vi "Read firmware file.vi"(2 "error in":errorcluster, 3 "RBF file path in":path) -> (0 "error out":errorcluster, 1 "firmware data":u8[](array[numeric]))   [LabVIEW 2013]
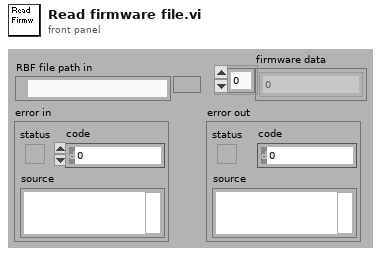
[diagram p1: front panel]
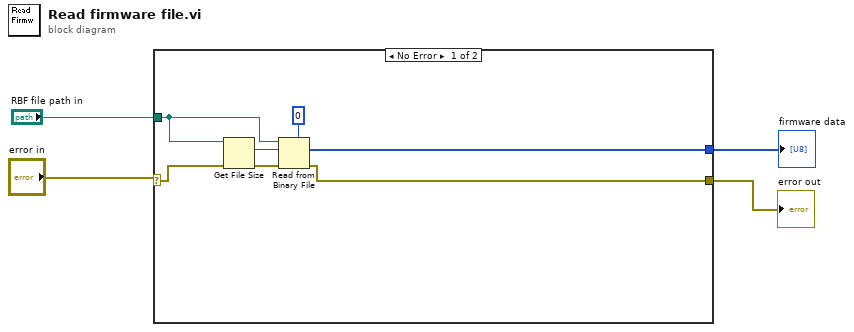
[diagram p0: block diagram]
diagram:
  n1 = case shown="No Error" "error in" {
    selector: "error in" -> [w11 w12]
    tunnel: "RBF file path in" -> [w8 _]
    tunnel: [w6 _] -> w1
    tunnel: [w5 w12] -> w2
    frame No Error {
      n2 = Get File Size(file=w8, error in=w11) -> (size (in bytes)=w9:i64, 0:w10:errorcluster)  [unwired: 1 out]
      n3 = Read from Binary File(5:u8 0, 8:w10, 10:w9, 11:w8) -> (0:w5:errorcluster, 2:w6:u8[])  [unwired: 4 out]
    }
    frame Error {
    }
  }
  "error out" <- w2
  "firmware data" <- w1
